vi "Set LED (PWM).vi"(8 "error in (no error)":errorcluster, 9 "PWM (0-255)":u8, 10 "LED Selector":T1, 11 "LINX-AutomationHat in":refnum<class "LINX-AutomationHat.lvclass">) -> (0 "error out":errorcluster, 3 "LINX-AutomationHat out":refnum<class "LINX-AutomationHat.lvclass">)   [LabVIEW 2020, in "LINX-AutomationHat.lvclass"]
doc: "Sets the LED PWM/brightness."
uses:
  LINX-AutomationHat.lvclass
  LEDs.ctl
  LINX-SN3218/LINX-SN3218.lvclass
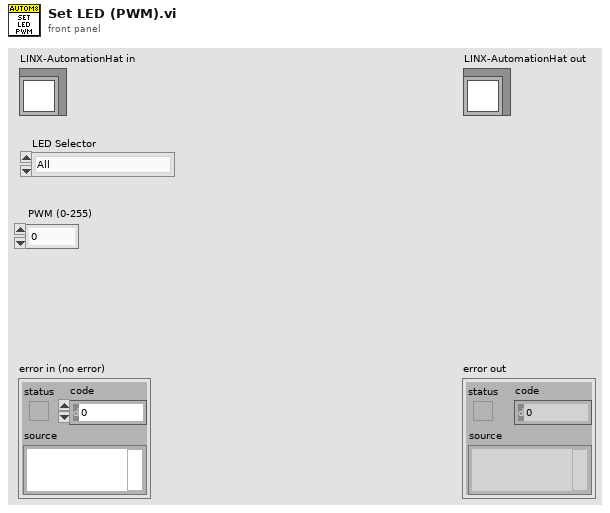
[diagram p1: front panel]
types:
  T1 = typedef "LINX-AutomationHat.lvclass/LEDs.ctl" = enum16{"All", "ADC1", "ADC2", "ADC3", "Output1", "Output2", "Output3", "Relay1NO", "Relay1NC", "Relay2NO", "Relay2NC", "Relay3NO", "Relay3NC", "Input3", "Input2", "Input1", "Warn", "Comms", "Power"}
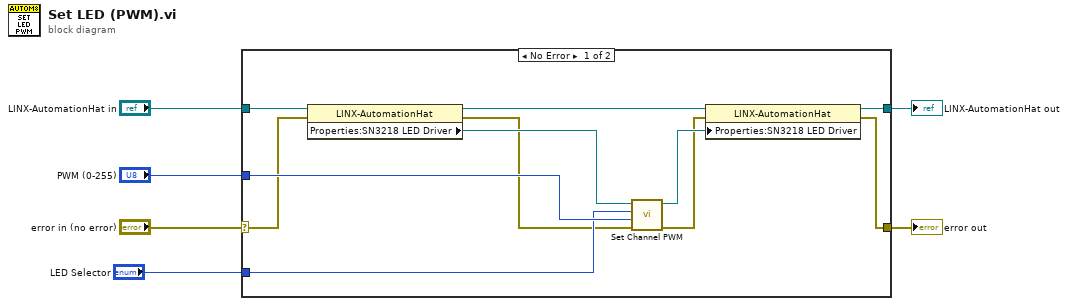
[diagram p0: block diagram]
diagram:
  n1 = case shown="No Error" "error in (no error)" {
    selector: "error in (no error)" -> [w8 w19]
    tunnel: [w9 w19] -> w5
    tunnel: [w12 w18] -> w3
    tunnel: "LINX-AutomationHat in" -> [w17 w18]
    tunnel: "PWM (0-255)" -> [w15 _]
    tunnel: "LED Selector" -> [w14 _]
    frame No Error {
      n2 = property class="LINX-AutomationHat"(reference=w17, error in=w8) -> (reference out=w13:refnum<class "LINX-AutomationHat.lvclass">, error out=w7:errorcluster, "Properties:SN3218 LED Driver"=w16:refnum<class "LINX-SN3218.lvclass">)
      n3 = call "Set Channel PWM.vi"("error in (no error)"=w7, "PWM (0-255)"=w15, "LED Channel (0-18, 0=all)"=w14, "LINX-SN3218 in"=w16) -> ("error out"=w10:errorcluster, "LINX-SN3218 out"=w11:refnum<class "LINX-SN3218.lvclass">)  [unwired: 6 in]
      n4 = property class="LINX-AutomationHat"(reference=w13, error in=w10, "Properties:SN3218 LED Driver"=w11) -> (reference out=w12:refnum<class "LINX-AutomationHat.lvclass">, error out=w9:errorcluster)
    }
    frame Error {
    }
  }
  "error out" <- w5
  "LINX-AutomationHat out" <- w3
